vi "DCS Waveform Analyzer.vi"(8 "Rank":i32=30, 11 "8 DCS Waveforms":dbl[][](array[numeric])) -> (0 "Filtered Signals":dbl[][](array[numeric]), 3 "Maxs":dbl[](array[numeric]))   [LabVIEW 2015]
doc: "Takes waveform as 2D array and \"rank\". Performs a median filter using \"rank\" as the window size. Also returns a 1D array of channel maxes."
uses:
  <vilib>/Analysis/NI_AALBase.lvlib
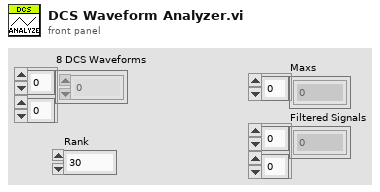
[diagram p1: front panel]
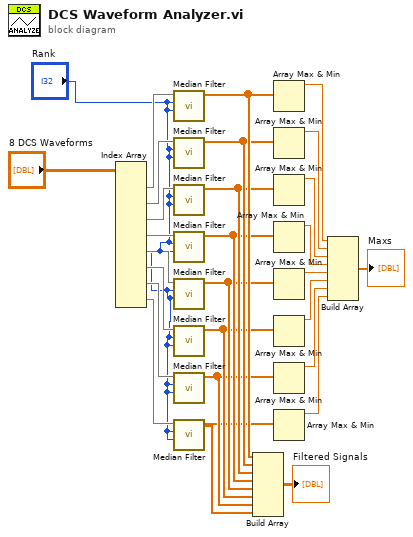
[diagram p0: block diagram]
diagram:
  n1 = Index Array(array="8 DCS Waveforms") -> (element #1=w28:dbl[], element #2=w27:dbl[], element #3=w26:dbl[], element #4=w25:dbl[], element #5=w24:dbl[], element #6=w23:dbl[], element #7=w22:dbl[], element #8=w21:dbl[])  [unwired: 16 in]
  n2 = call <vilib>:"Median Filter.vi"("right rank"="Rank", "left rank"="Rank", "X"=w28) -> ("Filtered X"=w18:dbl[])  [unwired: 7 in, 1 out]
  n3 = call <vilib>:"Median Filter.vi"("right rank"="Rank", "left rank"="Rank", "X"=w27) -> ("Filtered X"=w17:dbl[])  [unwired: 7 in, 1 out]
  n4 = call <vilib>:"Median Filter.vi"("right rank"="Rank", "left rank"="Rank", "X"=w26) -> ("Filtered X"=w16:dbl[])  [unwired: 7 in, 1 out]
  n5 = call <vilib>:"Median Filter.vi"("right rank"="Rank", "left rank"="Rank", "X"=w25) -> ("Filtered X"=w15:dbl[])  [unwired: 7 in, 1 out]
  n6 = call <vilib>:"Median Filter.vi"("right rank"="Rank", "left rank"="Rank", "X"=w24) -> ("Filtered X"=w14:dbl[])  [unwired: 7 in, 1 out]
  n7 = call <vilib>:"Median Filter.vi"("right rank"="Rank", "left rank"="Rank", "X"=w23) -> ("Filtered X"=w13:dbl[])  [unwired: 7 in, 1 out]
  n8 = call <vilib>:"Median Filter.vi"("right rank"="Rank", "left rank"="Rank", "X"=w22) -> ("Filtered X"=w12:dbl[])  [unwired: 7 in, 1 out]
  n9 = call <vilib>:"Median Filter.vi"("right rank"="Rank", "left rank"="Rank", "X"=w21) -> ("Filtered X"=w11:dbl[])  [unwired: 7 in, 1 out]
  n10 = Build Array(w18, w17, w16, w15, w14, w13, w12, w11) -> (→"Filtered Signals":dbl[][])
  n11 = Array Max & Min(array=w18) -> (max value=w10:dbl)  [unwired: 3 out]
  n12 = Array Max & Min(array=w17) -> (max value=w9:dbl)  [unwired: 3 out]
  n13 = Array Max & Min(array=w16) -> (max value=w8:dbl)  [unwired: 3 out]
  n14 = Array Max & Min(array=w15) -> (max value=w7:dbl)  [unwired: 3 out]
  n15 = Array Max & Min(array=w14) -> (max value=w6:dbl)  [unwired: 3 out]
  n16 = Array Max & Min(array=w13) -> (max value=w5:dbl)  [unwired: 3 out]
  n17 = Array Max & Min(array=w12) -> (max value=w4:dbl)  [unwired: 3 out]
  n18 = Array Max & Min(array=w11) -> (max value=w3:dbl)  [unwired: 3 out]
  n19 = Build Array(w10, w9, w8, w7, w6, w5, w4, w3) -> (→"Maxs":dbl[])
